vi "Setup.vi"(9 "Active Project":refnum<vi>, 10 "NI.LV.Dialog Instance":refnum<vi>) -> (2 "Target":string, 3 "_Template out":refnum<class "_Template.lvclass">)   [LabVIEW 2025, in "_Template.lvlib" / "_Template.lvclass"]
uses:
  _Template.lvclass
  _Template.lvclass/_Template.ctl
  _Shared/Project Stuff/Project Stuff.lvclass
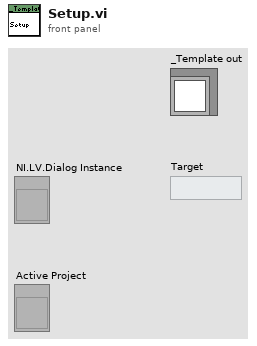
[diagram p1: front panel]
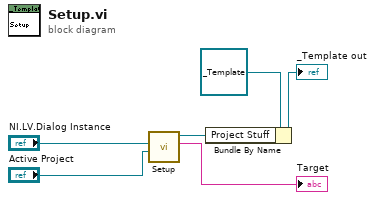
[diagram p0: block diagram]
diagram:
  n1 = call "Setup.vi"("Active Project"="Active Project", "NI.LV.Dialog Instance"="NI.LV.Dialog Instance") -> ("Target"=→"Target":string, "Project Stuff out"=w6:refnum<class "Project Stuff.lvclass">)  [unwired: 8 in]
  n2 = Bundle By Name(cluster=refnum<class "_Template.lvclass"> refnum ("_Create From Template.lvlib:Script Strategy.lvlib:First Library Script Strategy.lvclass"), "Project Stuff"=w6) -> (→"_Template out":refnum<class "_Template.lvclass">)
